vi "Magazine_Globals.vi"() -> ()   [LabVIEW 2019]
uses:
  Subsystems/Magazine/Magazine_Cluster.ctl
  Subsystems/Magazine/Magazine_States.ctl
panel:
  in  "Top_Middle_IR":string="Top_Middle_IR"
  in  "Bottom_Middle_IR":string="Bottom_Middle_IR"
  in  "Bottom_IR":string="Bottom_IR"
  in  "Top_IR":string="Top_IR"
  in  "Magazine":string="Magazine"
  in  "Magazine_Execute_Notifier":refnum<notifier>
  in  "Magazine_Set_Notifier":refnum<notifier>
  in  "Magazine_Execute_Ref":string="Magazine_Execute_Ref"
  in  "Magazine_Set_Ref":string="Magazine_Set_Ref"
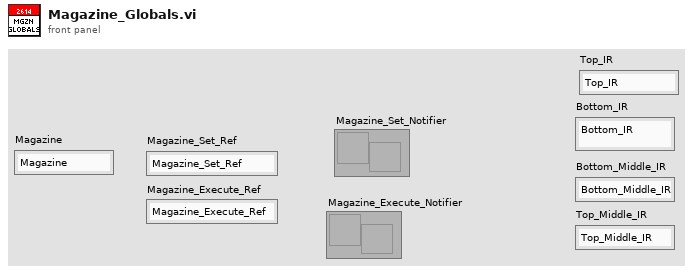
[diagram p1: front panel]
diagram:
